vi "Command.vi"(8 "error in (no error)":errorcluster, 11 "Node Ptr":T1 format="%.0x") -> (0 "error out":errorcluster)   [LabVIEW 2020, in "Instrument Addon System Explorer.lvlib"]
uses:
  Instrument Addon System Explorer.lvlib
  <vilib>/NI VeriStand/Custom Device API/Custom Device Item Ref.ctl
  Addon Shared/Types/FG Control.ctl
  Addon Shared/SubVIs/Constants.vi
  <vilib>/NI VeriStand/Custom Device API/NI VeriStand - Get Item Property.vi
  <vilib>/NI VeriStand/Custom Device API/Get Item Property (String).vi
  <vilib>/NI VeriStand/Custom Device API/Get Item Property (String Array).vi
  <vilib>/NI VeriStand/Custom Device API/Get Item Property (Boolean).vi
  <vilib>/NI VeriStand/Custom Device API/Get Item Property (U32).vi
  <vilib>/NI VeriStand/Custom Device API/NI VeriStand - Set Item Property.vi
  <vilib>/NI VeriStand/Custom Device API/Set Item Property (String).vi
  <vilib>/NI VeriStand/Custom Device API/Set Item Property (String Array).vi
  <vilib>/NI VeriStand/Custom Device API/Set Item Property (Boolean).vi
  <vilib>/NI VeriStand/Custom Device API/Set Item Property (U32).vi
  <vilib>/NI VeriStand/Custom Device API/Custom Device API.lvlib
  Addon Shared/Instrument Addon Shared.lvlib
panel:
  in  "Pad Value":u8=32 format="%.0x"
  in  "Length":u32=25 caption="Length (Bytes)"
  in  "Pad":bool caption="Pad?"
  in  "Linkages":i32(listbox)
  in  "MetaData":string(combo) caption="Available MetaData Channels"
  in  "Command":string caption="Command ( Use [] to define a variable )"
  in  "Header 2":cluster{"Section Name":string}={"Section Name"="Command Message Settings"}
  in  "SHDocVw.IWebBrowser":refnum<k7>(container)
  in  "Header":cluster{"Section Name":string}={"Section Name"="Command Settings"}
  in  "Description":string
  out "Name":string
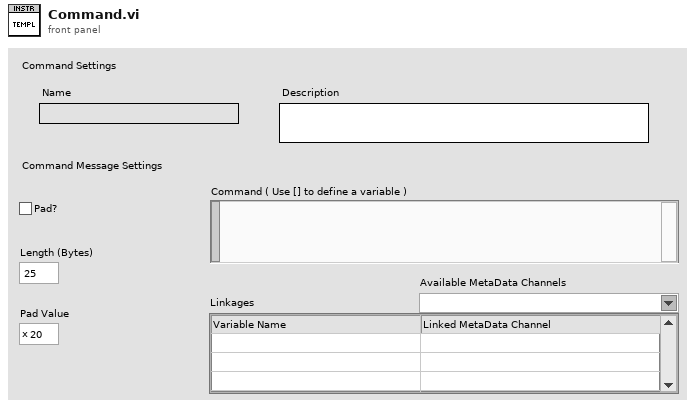
[diagram p1: front panel]
types:
  T1 = typedef "Custom Device API.lvlib/Custom Device Item Ref.ctl" = u64
  T2 = typedef "Instrument Addon Shared.lvlib/FG Control.ctl" = enum16{"Get", "Set"}
  T3 = typedef "Instrument Addon Shared.lvlib/Command Parameters.ctl" = cluster{"Command":string, "Linked Channels":T4[], "Pad":bool, "Length":u32, "Pad Value":u8}
  T4 = typedef "Instrument Addon Shared.lvlib/Linked Channel Cluster.ctl" = cluster{"Variable Name":string, "GUID":string}
  T5 = typedef "Custom Device API.lvlib/Custom Device Item Info.ctl" = cluster{"Name":string, "Is Channel":bool, "GUID":string, "Is Waveform":bool}
  T6 = typedef "Custom Device API.lvlib/Custom Device Commands.ctl" = enum16{"Default", "Item renamed", "Shutdown", "Dynamic button pressed"}
  T7 = typedef "LVComboBoxStrsAndValuesArrayTypeDef.ctl" = cluster{"String":string, "Value":string}[]
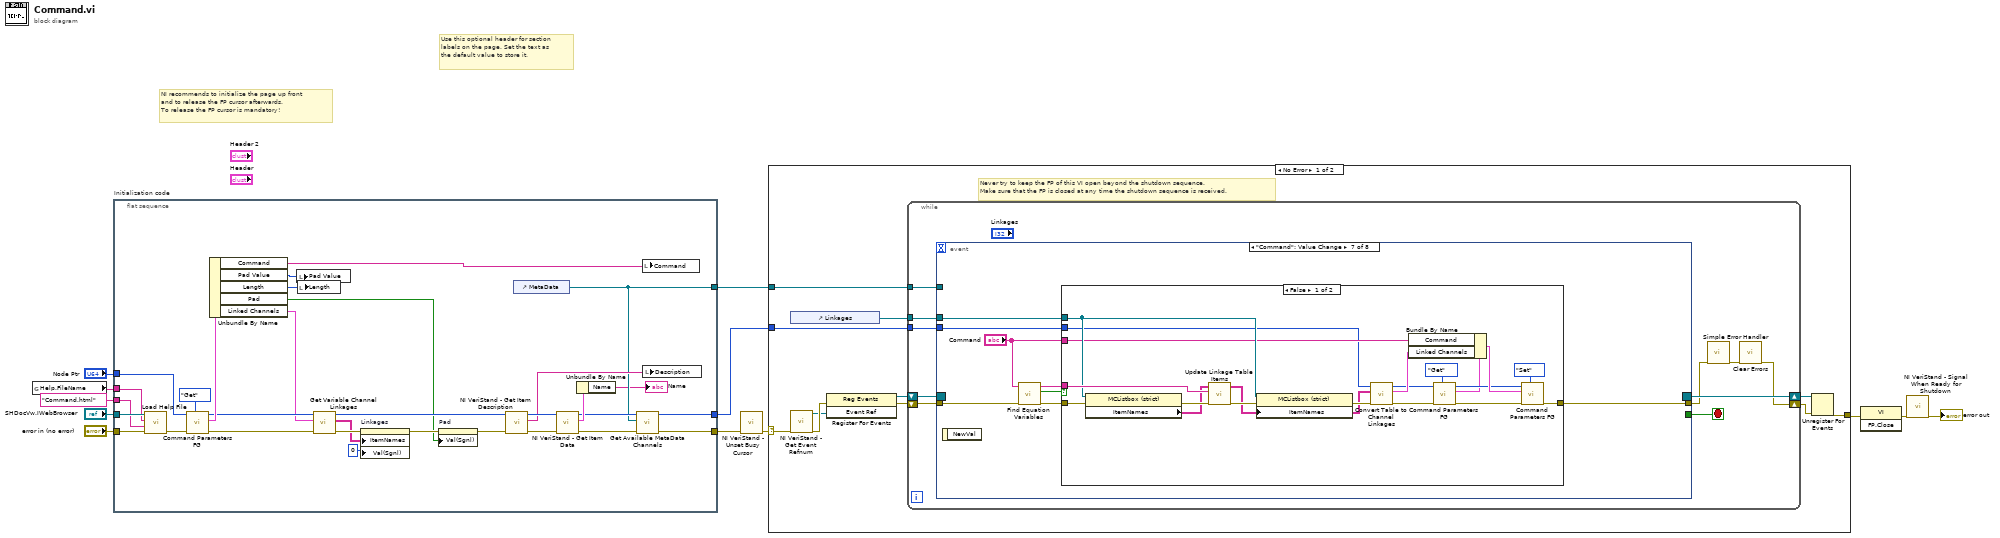
[diagram p0: block diagram]
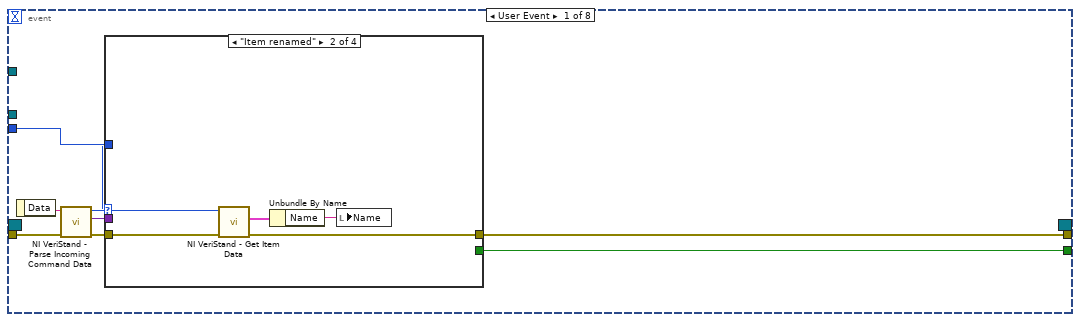
[diagram p2: hidden frame]
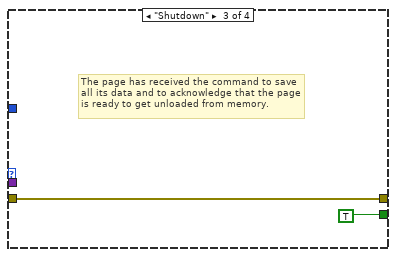
[diagram p4: hidden frame]
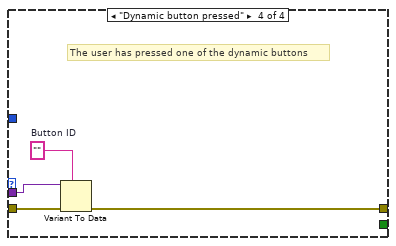
[diagram p5: hidden frame]
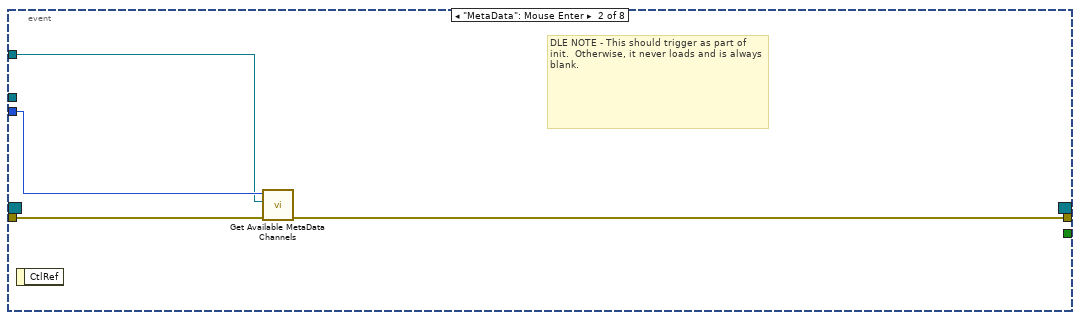
[diagram p6: hidden frame]
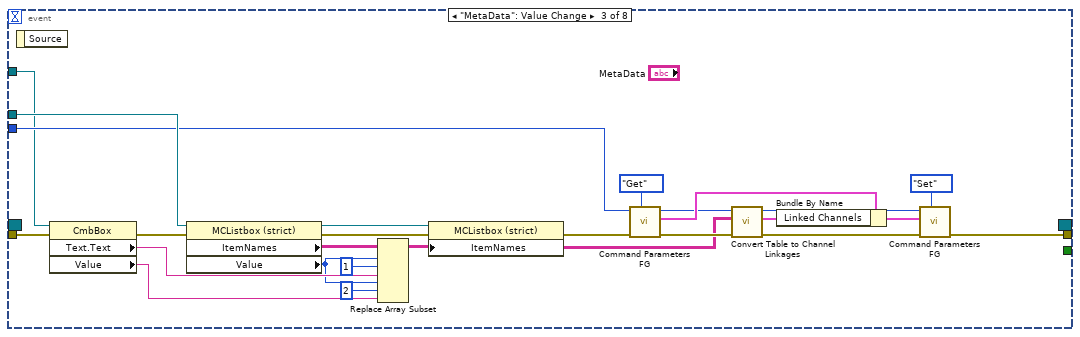
[diagram p7: hidden frame]
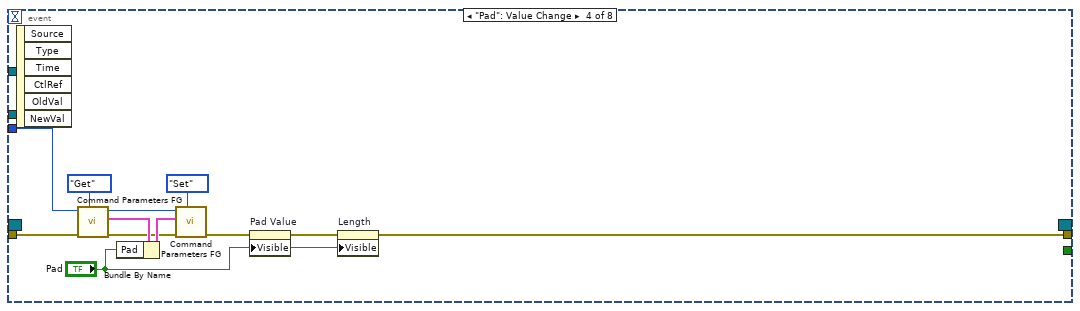
[diagram p8: hidden frame]
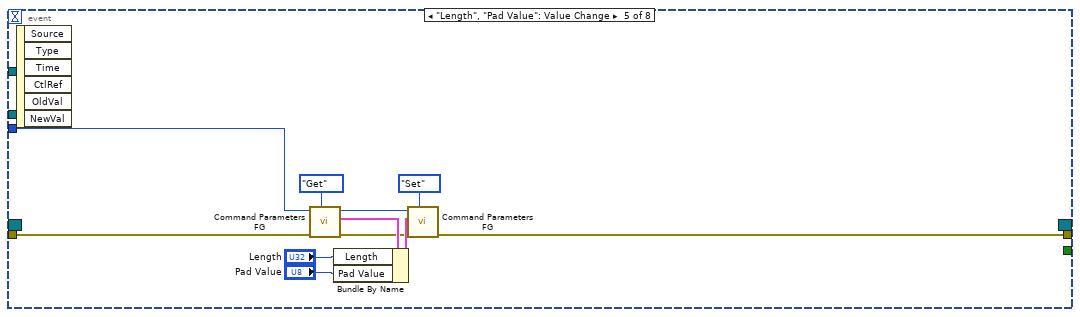
[diagram p9: hidden frame]
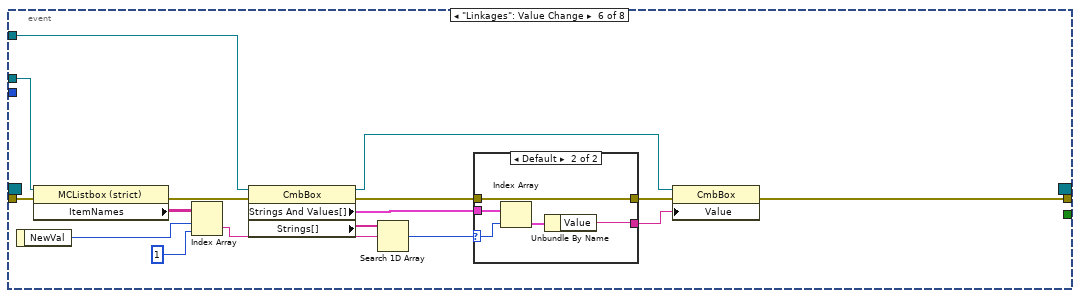
[diagram p10: hidden frame]
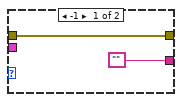
[diagram p11: hidden frame]
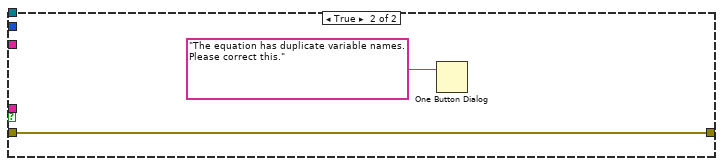
[diagram p12: hidden frame]
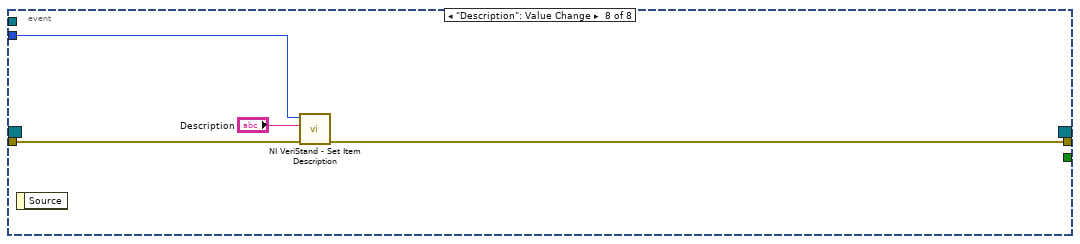
[diagram p13: hidden frame]
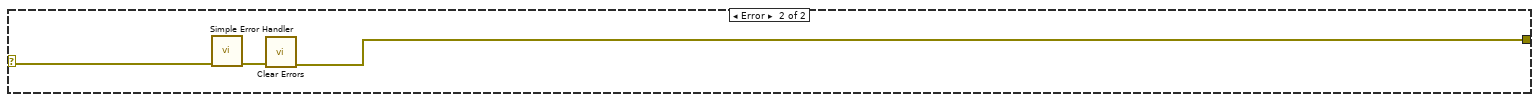
[diagram p14: hidden frame]
diagram:
  # "Use this optional header for section labels on the page. Set the text as the default value to store it."
  # "NI recommends to initialize the page up front\nand to release the FP cursor afterwards.\nTo release the FP cursor is mandatory!"
  n1 = global read "Constants.vi" "Help.FileName"() -> (w1:string)
  n2 = flat-sequence "Initialization code" {
    tunnel: "error in (no error)" -> [w39]
    tunnel: "Node Ptr" -> [w34]
    tunnel: [w28] -> w8
    tunnel: [w26] -> w5
    tunnel: "SHDocVw.IWebBrowser" -> [w38]
    tunnel: "Command.html" ("HTML File") -> [w37]
    tunnel: w1 -> [w36]
    tunnel: [w25] -> w2
    frame #0 {
      n3 = call "Load Help File.vi"("error in (no error)"=w39, "HTML File"=w37, "Main CHM File"=w36, "SHDocVw.IWebBrowser2"=w38) -> ("error out"=w33:errorcluster)  [unwired: 7 in]
      n4 = call "Command Parameters FG.vi"("Action"=FG_Control."Get", "error in (no error)"=w33, "Item Ref in"=w34) -> ("error out"=w23:errorcluster, "Command Parameters"=w32:T3, "Item Ref out"=w22:T1)  [unwired: 6 in]
      n5 = Unbundle By Name(w32) -> ("Command"=w31:string, "Pad Value"=w14:u8, "Length"=w13:u32, "Pad"=w15:bool, "Linked Channels"=w21:T4[])
      n6 = local write "Pad Value"(w14) -> ()
      n7 = local write "Length"(w13) -> ()
      n8 = call "Get Variable Channel Linkages.vi"("error in (no error)"=w23, "Linked Channels"=w21, "Item Ref in"=w22) -> ("error out"=w20:errorcluster, "Array"=w19:string[][], "Item Ref out"=w18:T1)  [unwired: 6 in]
      n9 = property on="Linkages" class="MCListbox (strict)"(error in=w20, "ItemNames"=w19, "Val(Sgnl)"=0 ("Value (Signaling)")) -> (error out=w17:errorcluster)  [unwired: 1 in, 1 out]
      n10 = property on="Pad" class="Bool (strict)"(error in=w17, "Val(Sgnl)"=w15) -> (error out=w16:errorcluster)  [unwired: 1 in, 1 out]
      n11 = call <vilib>:"NI VeriStand - Get Item Description.vi"("error in (no error)"=w16, "Item Ref in"=w18) -> ("error out"=w41:errorcluster, "Description"=w42:string, "Item Ref out"=w43:T1)  [unwired: 7 out]
      n12 = control-ref of="MetaData"() -> (w25:refnum<vi>)
      n13 = call <vilib>:"NI VeriStand - Get Item Data.vi"("error in (no error)"=w41, "Item Ref in"=w43) -> ("error out"=w29:errorcluster, "Item Info"=w40:T5, "Item Ref out"=w27:T1)  [unwired: 7 out]
      n14 = Unbundle By Name(w40) -> ("Name"=→"Name":string)
      n15 = call "Get Available MetaData Channels.vi"("error in (no error)"=w29, "MetaData"=w25, "Item Ref in"=w27) -> ("error out"=w28:errorcluster, "Item Ref out"=w26:T1)  [unwired: 7 in]
      n16 = local write "Command"(w31) -> ()
      n17 = local write "Description"(w42) -> ()
    }
  }
  n18 = call <vilib>:"NI VeriStand - Unset Busy Cursor.vi"("error in (no error)"=w8) -> ("error out"=w7:errorcluster)  [unwired: 10 out]
  n19 = case shown="No Error" w7 {
    selector: w7 -> [w46 w196]
    tunnel: [w51 w194] -> w12
    tunnel: w5 -> [w47 _]
    tunnel: w2 -> [w44 _]
    frame No Error {
      # "Never try to keep the FP of this VI open beyond the shutdown sequence.\nMake sure that the FP is closed at any time the shutdown sequence is received."
      n20 = call <vilib>:"NI VeriStand - Get Event Refnum.vi"("error in (no error)"=w46) -> ("error out"=w54:errorcluster, "Event Ref"=w50:refnum<user-event>)  [unwired: 9 out]
      n21 = control-ref of="Linkages"() -> (w45:refnum<vi>)
      n22 = register-events(error in=w54, w50) -> (reference out=w48:refnum<event-registration>, error out=w49:errorcluster)  [unwired: 1 in]
      n23 = while {
        tunnel: w47 -> [w56]
        shift-right: [w59] -> w52
        shift-left: w49 -> [w63]
        shift-right: [w64] -> w53
        shift-left: w48 -> [w62]
        tunnel: w45 -> [w58]
        tunnel: w44 -> [w57]
        stop <- w61 stop-if-true
        n24 = event shown="[6] \"Command\": Value Change" {
          selector: w62 -> [_ _ _ _ _ _ _ _]
          dyn-events: [_ _ _ _ _ _ _ _] -> w64
          timeout: _ -> [_ _ _ _ _ _ _ _]
          tunnel: w63 -> [w72 w88 w97 w120 w131 w152 w166 w192]
          tunnel: [w68 _ _ _ _ _ _ _] -> w61
          tunnel: [w67 w87 w105 w115 w128 w142 w163 w191] -> w55
          tunnel: w58 -> [_ _ w113 _ _ w151 w164 _]
          tunnel: w57 -> [_ w85 w98 _ _ w147 _ _]
          tunnel: w56 -> [w66 w86 w101 w122 w133 _ w161 w193]
          event User Event {
            n25 = event-data() -> ("Data"=w71:string)  [unwired: 1 out]
            n26 = call <vilib>:"NI VeriStand - Parse Incoming Command Data.vi"("error in (no error)"=w72, "Incoming data"=w71) -> ("error out"=w70:errorcluster, "Outgoing data"=w65:variant, "Action"=w69:T6)  [unwired: 7 out]
            n27 = case shown="\"Item renamed\"" w69 {
              tunnel: w70 -> [w73 w78 w79 w84]
              tunnel: [_ _ TRUE _] -> w68
              tunnel: [w73 w75 w79 w81] -> w67
              tunnel: w66 -> [_ w77 _ _]
              tunnel: w65 -> [_ _ _ w83]
              frame "Default", Default {
              }
              frame "Item renamed" {
                n28 = call <vilib>:"NI VeriStand - Get Item Data.vi"("error in (no error)"=w78, "Item Ref in"=w77) -> ("error out"=w75:errorcluster, "Item Info"=w76:T5)  [unwired: 8 out]
                n29 = Unbundle By Name(w76) -> ("Name"=w74:string)
                n30 = local write "Name"(w74) -> ()
              }
              frame "Shutdown" {
                # "The page has received the command to save all its data and to acknowledge that the page is ready to get unloaded from memory."
              }
              frame "Dynamic button pressed" {
                w82 = ""  # Button ID
                # "The user has pressed one of the dynamic buttons"
                n31 = Variant To Data(error in=w84, type=w82, Variant=w83) -> (error out=w81:errorcluster)  [unwired: 1 out]
              }
            }
          }
          event "MetaData": Mouse Enter {
            # "DLE NOTE - This should trigger as part of init.  Otherwise, it never loads and is always blank."
            n32 = event-data() -> ()  [unwired: 2 out]
            n33 = call "Get Available MetaData Channels.vi"("error in (no error)"=w88, "MetaData"=w85, "Item Ref in"=w86) -> ("error out"=w87:errorcluster)  [unwired: 7 in, 1 out]
          }
          event "MetaData": Value Change {
            n34 = event-data() -> ()  [unwired: 2 out]
            n35 = property class="CmbBox"(reference=w98, error in=w97) -> (error out=w96:errorcluster, "Text.Text"=w95:string, "Value"=w93:string)  [unwired: 1 out]
            n36 = property class="MCListbox (strict)"(reference=w113, error in=w96) -> (reference out=w110:refnum<vi>, error out=w109:errorcluster, "ItemNames"=w112:string[][], "Value"=w94:i32)
            n37 = Replace Array Subset(array=w112, new element #1=w95, index (row) #1=w94, index (col) #1=1 ("disabled index (col)"), new element #2=w93, index (row) #2=w94, index (col) #2=2 ("disabled index (col)")) -> (w92:string[][])
            n38 = property class="MCListbox (strict)"(reference=w110, error in=w109, "ItemNames"=w92) -> (error out=w103:errorcluster)  [unwired: 1 out]
            n39 = call "Command Parameters FG.vi"("Action"=FG_Control."Get", "error in (no error)"=w103, "Item Ref in"=w101) -> ("error out"=w102:errorcluster, "Command Parameters"=w100:T3, "Item Ref out"=w90:T1)  [unwired: 6 in]
            n40 = call "Convert Table to Channel Linkages.vi"("error in (no error)"=w102, "Item Names"=w92, "Item Ref in"=w90) -> ("error out"=w107:errorcluster, "Linkages"=w91:T4[], "Item Ref out"=w89:T1)  [unwired: 6 in]
            n41 = Bundle By Name(cluster=w100, "Linked Channels"=w91) -> (w106:T3)
            n42 = call "Command Parameters FG.vi"("Action"=FG_Control."Set", "error in (no error)"=w107, "Command Parameters"=w106, "Item Ref in"=w89) -> ("error out"=w105:errorcluster)  [unwired: 5 in, 2 out]
          }
          event "Pad": Value Change {
            n43 = event-data() -> ()  [unwired: 7 out]
            n44 = call "Command Parameters FG.vi"("Action"=FG_Control."Get", "error in (no error)"=w120, "Item Ref in"=w122) -> ("error out"=w119:errorcluster, "Command Parameters"=w121:T3, "Item Ref out"=w118:T1)  [unwired: 6 in]
            n45 = Bundle By Name(cluster=w121, "Pad"="Pad") -> (w124:T3)
            n46 = call "Command Parameters FG.vi"("Action"=FG_Control."Set", "error in (no error)"=w119, "Command Parameters"=w124, "Item Ref in"=w118) -> ("error out"=w116:errorcluster)  [unwired: 5 in, 2 out]
            n47 = property on="Pad Value" class="DigNum (strict)"(error in=w116, "Visible"="Pad") -> (error out=w117:errorcluster)  [unwired: 1 in, 1 out]
            n48 = property on="Length" class="DigNum (strict)"(error in=w117, "Visible"="Pad") -> (error out=w115:errorcluster)  [unwired: 1 in, 1 out]
          }
          event "Length", "Pad Value": Value Change {
            n49 = event-data() -> ()  [unwired: 7 out]
            n50 = call "Command Parameters FG.vi"("Action"=FG_Control."Get", "error in (no error)"=w131, "Item Ref in"=w133) -> ("error out"=w130:errorcluster, "Command Parameters"=w132:T3, "Item Ref out"=w129:T1)  [unwired: 6 in]
            n51 = Bundle By Name(cluster=w132, "Length"="Length", "Pad Value"="Pad Value") -> (w135:T3)
            n52 = call "Command Parameters FG.vi"("Action"=FG_Control."Set", "error in (no error)"=w130, "Command Parameters"=w135, "Item Ref in"=w129) -> ("error out"=w128:errorcluster)  [unwired: 5 in, 2 out]
          }
          event "Linkages": Value Change {
            n53 = event-data() -> ("NewVal"=w149:i32)  [unwired: 1 out]
            n54 = property class="MCListbox (strict)"(reference=w151, error in=w152) -> (error out=w146:errorcluster, "ItemNames"=w150:string[][])  [unwired: 1 out]
            n55 = Index Array(array=w150, index (row)=w149, index (col)=1 ("disabled index (col)")) -> (element=w145:string)
            n56 = property class="CmbBox"(reference=w147, error in=w146) -> (reference out=w140:refnum<vi>, error out=w138:errorcluster, "Strings And Values[]"=w144:T7, "Strings[]"=w137:string[])
            n57 = Search 1D Array(1D array=w137, element=w145) -> (index of element=w141:i32)  [unwired: 1 in]
            n58 = case shown="Default" w141 {
              selector: w141 -> [_ w157]
              tunnel: w144 -> [_ w159]
              tunnel: ["" w155] -> w143
              tunnel: [w154 w156] -> w139
              tunnel: w138 -> [w154 w156]
              frame -1 {
              }
              frame Default {
                n59 = Index Array(array=w159, index=w157) -> (element=w158:cluster{"String":string, "Value":string})
                n60 = Unbundle By Name(w158) -> ("Value"=w155:string)
              }
            }
            n61 = property class="CmbBox"(reference=w140, error in=w139, "Value"=w143) -> (error out=w142:errorcluster)  [unwired: 1 out]
          }
          event "Command": Value Change {
            n62 = event-data() -> ()  [unwired: 2 out]
            n63 = call "Find Equation Variables.vi"("error in (no error)"=w166, "Command"="Command") -> ("error out"=w165:errorcluster, "Duplicate?"=w160:bool, "Variables"=w167:string[])  [unwired: 7 in]
            n64 = case shown="False" w160 {
              tunnel: w167 -> [w187 _]
              tunnel: w165 -> [w186 w189]
              tunnel: w164 -> [w182 _]
              tunnel: [w181 w189] -> w163
              tunnel: "Command" -> [w180 _]
              tunnel: w161 -> [w174 _]
              frame False {
                n65 = property class="MCListbox (strict)"(reference=w182, error in=w186) -> (error out=w185:errorcluster, "ItemNames"=w184:string[][])  [unwired: 1 out]
                n66 = call "Update Linkage Table Items.vi"("error in (no error)"=w185, "Variables"=w187, "Item Names"=w184) -> ("error out"=w183:errorcluster, "Item Names"=w176:string[][])  [unwired: 7 in]
                n67 = property class="MCListbox (strict)"(reference=w182, error in=w183, "ItemNames"=w176) -> (error out=w178:errorcluster)  [unwired: 1 out]
                n68 = call "Convert Table to Channel Linkages.vi"("error in (no error)"=w178, "Item Names"=w176, "Item Ref in"=w174) -> ("error out"=w172:errorcluster, "Linkages"=w175:T4[], "Item Ref out"=w170:T1)  [unwired: 6 in]
                n69 = call "Command Parameters FG.vi"("Action"=FG_Control."Get", "error in (no error)"=w172, "Item Ref in"=w170) -> ("error out"=w171:errorcluster, "Command Parameters"=w168:T3, "Item Ref out"=w169:T1)  [unwired: 6 in]
                n70 = Bundle By Name(cluster=w168, "Command"=w180, "Linked Channels"=w175) -> (w177:T3)
                n71 = call "Command Parameters FG.vi"("Action"=FG_Control."Set", "error in (no error)"=w171, "Command Parameters"=w177, "Item Ref in"=w169) -> ("error out"=w181:errorcluster)  [unwired: 5 in, 2 out]
              }
              frame True {
                n72 = One Button Dialog(message="The equation has duplicate variable names.  Please correct this.") -> ()  [unwired: 1 in, 1 out]
              }
            }
          }
          event "Description": Value Change {
            n73 = event-data() -> ()  [unwired: 2 out]
            n74 = call <vilib>:"NI VeriStand - Set Item Description.vi"("error in (no error)"=w192, "Description"="Description", "Item Ref in"=w193) -> ("error out"=w191:errorcluster)  [unwired: 8 out]
          }
        }
        n75 = call <vilib>:"Simple Error Handler.vi"("error in (no error)"=w55) -> ("error out"=w60:errorcluster)  [unwired: 1 in, 7 out]
        n76 = call <vilib>:"Clear Errors.vi"("error in (no error)"=w60) -> ("error out"=w59:errorcluster)  [unwired: 1 in, 5 out]
      }
      n77 = Unregister For Events(event registration refnum=w53, error in=w52) -> (error out=w51:errorcluster)
    }
    frame Error {
      n78 = call <vilib>:"Simple Error Handler.vi"("error in (no error)"=w196) -> ("error out"=w195:errorcluster)  [unwired: 1 in, 7 out]
      n79 = call <vilib>:"Clear Errors.vi"("error in (no error)"=w195) -> ("error out"=w194:errorcluster)  [unwired: 1 in, 5 out]
    }
  }
  n80 = invoke class="VI" method="FP.Close"(error in=w12) -> (error out=w11:errorcluster)  [unwired: 2 in, 2 out]
  n81 = call <vilib>:"NI VeriStand - Signal When Ready for Shutdown.vi"("error in (no error)"=w11) -> ("error out"=→"error out":errorcluster)  [unwired: 10 out]
